vi "Remaining_s.vi"(7 "Time period target":dbl caption="Time period target [s]", 11 "Error in":errorcluster caption="Error in (no error)", 12 "Start time in":i64=-1 caption="Start time in (-1: init) [ms]" min=-1 max=4294967295) -> (8 "Remaining time":dbl caption="Remaining time [s]", 10 "Elapsed time":dbl caption="Elapsed time [s]", 13 "Now":i64 caption="Now [ms]", 14 "Start time out":i64 caption="Start time out [ms]", 15 "Error out":errorcluster)   [LabVIEW 2017, in "GPTiming.lvlib"]
doc: "Calculates <B>Remaining time</B> of <B>Time period target</B> since <B>Start time in</B>.\n\n<B>Start time in</B> will be returned in <B>Start time out</B>. Set <B>Start time in</B> to -1 (or leave it unwired) to get the current time returned in <B>Start time out</B> instead. <B>Now</B> will always be the current time.\n\nThis VI uses the ms tick counter and will be able to count for 2^32-1 ms (almost 50 days) before <B>Remaining time</B> wraps around and starts over. <B>Remaining time</B> will be latched at 0 from when the remaining time runs out and until the tick counter wraps around. <B>Elapsed time</B> will continue counting up past the remaining time running out, thus you can use this output to see how late you were if you overshoot the <B>Time period target</B>.\n\nThis VI is inlined. <B>Error in</B> is wired straight through to <B>Error out</B> to enable optional dataflow dependency (offering control of when <B>Now</B> is).\n\nSteen Schmidt\nGPower\n8/12 2013"
uses:
  GPTiming.lvlib
panel:
  # "Copyright © 2013\nGPower\nSee enclosed license file for terms and conditions"
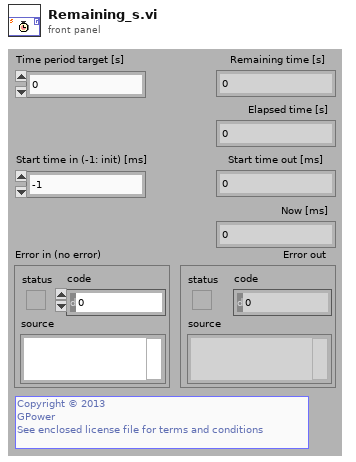
[diagram p1: front panel]
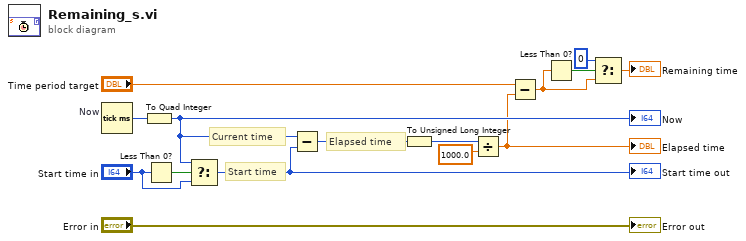
[diagram p0: block diagram]
diagram:
  # "Elapsed time"
  # "Current time"
  # "Start time"
  n1 = Tick Count (ms) "Now"() -> (millisecond timer value=w13:u32)
  n2 = To Quad Integer(1:w13) -> (0:w10:i64)
  "Now" <- w10
  n3 = Less Than 0?(x="Start time in") -> (x < 0?=w14:bool)
  n4 = Select(t=w10, s=w14, f="Start time in") -> (s? t:f=w11:i64)
  "Start time out" <- w11
  n5 = Subtract(x=w10, y=w11) -> (x-y=w9:i64)
  n6 = To Unsigned Long Integer(number=w9) -> (unsigned 32bit integer=w3:u32)
  n7 = Divide(x=w3, y=1000.0) -> (x/y=w2:dbl)
  "Elapsed time" <- w2
  n8 = Subtract(x="Time period target", y=w2) -> (x-y=w5:dbl)
  n9 = Less Than 0?(x=w5) -> (x < 0?=w6:bool)
  n10 = Select(t=u32 0, s=w6, f=w5) -> (s? t:f=→"Remaining time":dbl)
  "Error out" <- "Error in"
